vi "GET_Save_Layers_with_VI.vi"(8 "error in (no error)":errorcluster {"code" min=0 max=0}, 11 "Settings.lvclass in":refnum<class "Settings.lvclass">) -> (0 "error out":errorcluster {"code" min=0 max=0}, 2 "Merge user layers on commit":bool, 3 "Settings.lvclass out":refnum<class "Settings.lvclass">)   [LabVIEW 2020, in "Settings.lvclass"]
uses:
  Settings.lvclass
  Settings.lvclass/Settings.ctl
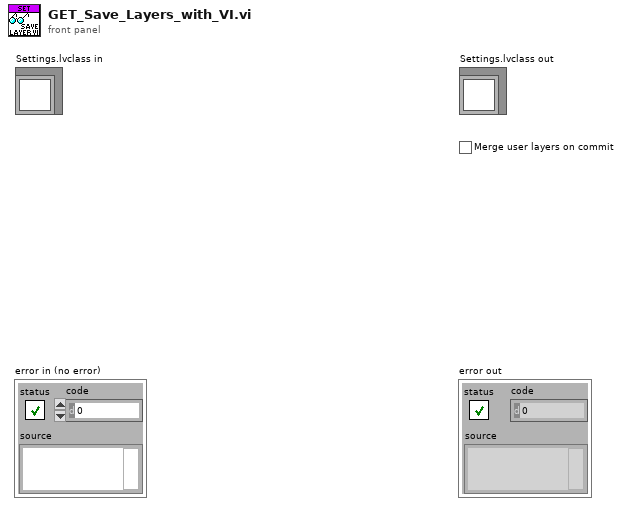
[diagram p1: front panel]
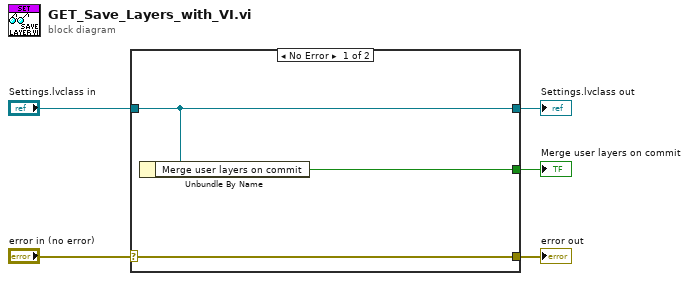
[diagram p0: block diagram]
diagram:
  n1 = case shown="No Error" "error in (no error)" {
    selector: "error in (no error)" -> [w8 w9]
    tunnel: [w8 w9] -> w4
    tunnel: [w7 w10] -> w2
    tunnel: "Settings.lvclass in" -> [w7 w10]
    tunnel: [w6 _] -> w1
    frame No Error {
      n2 = Unbundle By Name(w7) -> ("Merge user layers on commit"=w6:bool)
    }
    frame Error {
    }
  }
  "error out" <- w4
  "Settings.lvclass out" <- w2
  "Merge user layers on commit" <- w1
